vi "Cal Standard Instance.vi"(0 "Cal Standard Base in":refnum<class "Cal Standard Base.lvclass">, 5 "Operation":enum16{"Read", "Write", "Clear"}(ring), 11 "error in (no error)":errorcluster) -> (4 "Cal Standard Base out":refnum<class "Cal Standard Base.lvclass">, 6 "Found?":bool, 15 "error out":errorcluster)   [LabVIEW 2023, in "RFFixtureCharact.Instruments.lvlib" / "Cal Standard Factory.lvclass"]
uses:
  Cal Standard Factory.lvclass
  Cal Standard Base/Cal Standard Base.lvclass
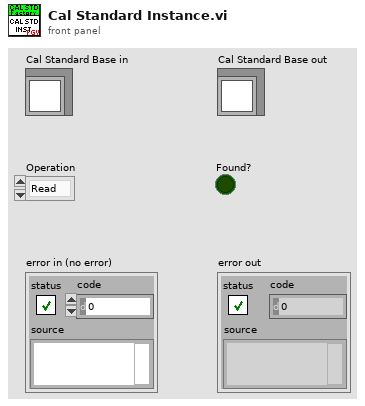
[diagram p1: front panel]
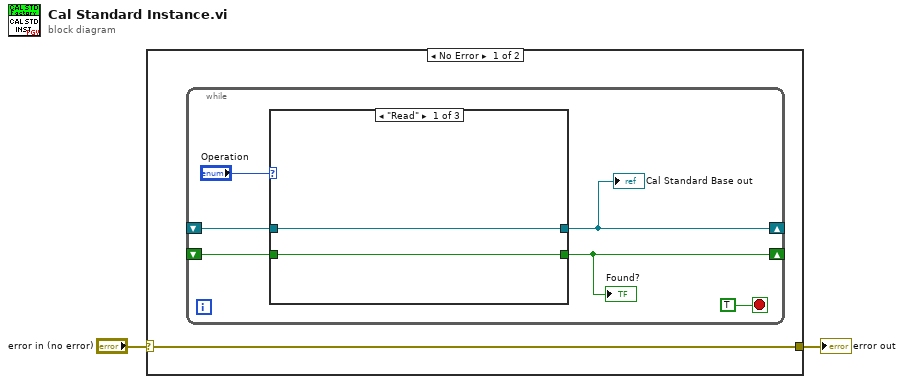
[diagram p0: block diagram]
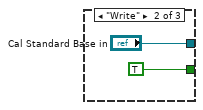
[diagram p2: hidden frame]
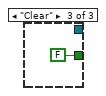
[diagram p3: hidden frame]
diagram:
  n1 = case shown="No Error" "error in (no error)" {
    selector: "error in (no error)" -> [w3 w15]
    tunnel: [w3 w15] -> w2
    frame No Error {
      n2 = while {
        shift-right: [w4] -> _
        shift-left: _ -> [w7]
        shift-right: [w6] -> _
        shift-left: _ -> [w5]
        stop <- TRUE stop-if-true
        n3 = case shown="\"Read\"" "Operation" {
          tunnel: [w11 "Cal Standard Base in" _] -> w4
          tunnel: w7 -> [w11 _ _]
          tunnel: [w10 TRUE FALSE] -> w6
          tunnel: w5 -> [w10 _ _]
          frame "Read" {
          }
          frame "Write" {
          }
          frame "Clear" {
          }
        }
        "Found?" <- w6
        "Cal Standard Base out" <- w4
      }
    }
    frame Error {
    }
  }
  "error out" <- w2
